vi "SimpleTest.vi"() -> ()   [LabVIEW 2010]
uses:
  <vilib>/NXT/Dual Mode Library/Display/drawNumber.vi
  <vilib>/NXT/Dual Mode Library/Waits/Wait_Num.vi
panel:
  out "value":i32
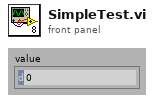
[diagram p1: front panel]
types:
  T1 = typedef "LVHSConnector.ctl" = cluster{"Hardware":string, "Flattened String":string}
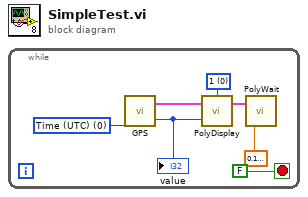
[diagram p0: block diagram]
diagram:
  n1 = while {
    stop <- FALSE stop-if-true
    w4 = i16 0 items=["1", "2", "3", "4", "5", "6", "7", "8"] ("Line")
    w7 = u16 0 items=["Time (UTC)"=0, "Status"=1, "Latitude"=2, "Longitude"=4, "Velocity (cm/s)"=6, "Heading (degrees)"=7, "Dist to destination (m)"=8, "Angle to destination (degrees)"=9, "Angle since last req"=10, "Set Destination Latitude"=11, "Set Destination Longitude"=12] ("Data Requested")
    n2 = call "GPS.vi"("Data Requested"=w7) -> ("value"=w5:i32, "NXT"=w6:T1)  [unwired: 2 in]
    "value" <- w5
    n3 = call-poly <vilib>:"PolyDisplay.vi"("number"=w5, "NXT"=w6, "Line"=w4) -> ("NXT"=w2:T1)  [unwired: 1 in]
    n4 = call-poly <vilib>:"PolyWait.vi"("Time (1 sec)"=sgl 0.1, "NXT"=w2) -> ()  [unwired: 2 in, 1 out]
  }
